vi "create_node.vi"(0 "text":string, 5 "metadatas":cluster{"key":string, "value":string}[](array[cluster]), 7 "vector":dbl[](array[numeric]), 11 "error in":errorcluster) -> (4 "data_node out":refnum<class "data_node.lvclass">, 15 "error out":errorcluster)   [LabVIEW 2020, in "data_node.lvclass"]
uses:
  data_node.lvclass
  data_node.lvclass/data_node.ctl
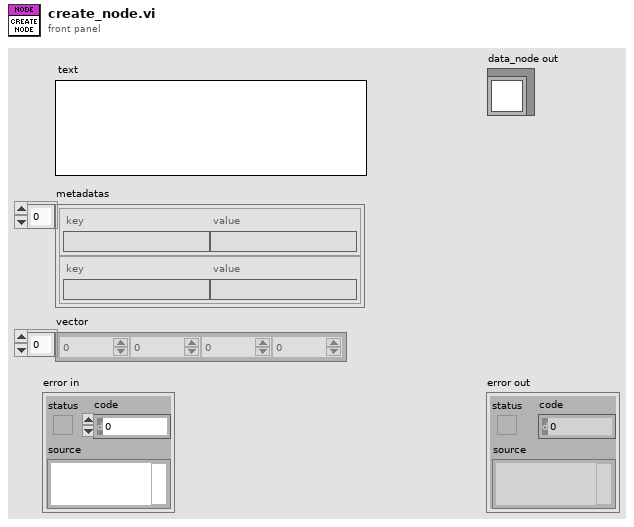
[diagram p1: front panel]
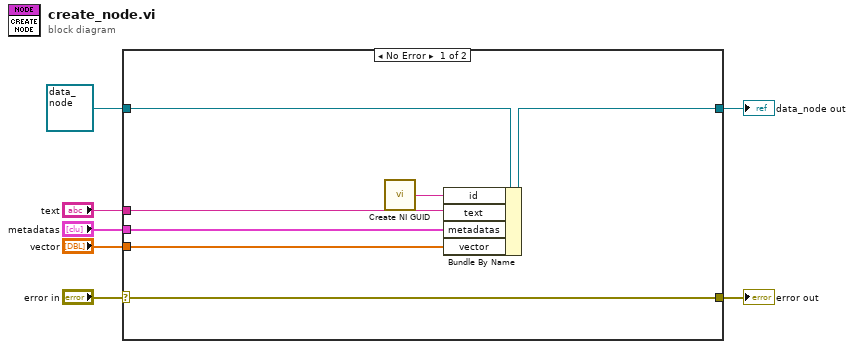
[diagram p0: block diagram]
diagram:
  n1 = case shown="No Error" "error in" {
    selector: "error in" -> [w14 w16]
    tunnel: [w14 w16] -> w6
    tunnel: [w11 w15] -> w4
    tunnel: refnum<class "data_node.lvclass"> refnum ("data_node in") -> [w13 w15]
    tunnel: "text" -> [w10 _]
    tunnel: "metadatas" -> [w9 _]
    tunnel: "vector" -> [w8 _]
    frame No Error {
      n2 = call <vilib>:"Create NI GUID.vi"() -> ("NI GUID"=w12:string)
      n3 = Bundle By Name(cluster=w13, "id"=w12, "text"=w10, "metadatas"=w9, "vector"=w8) -> (w11:refnum<class "data_node.lvclass">)
    }
    frame Error {
    }
  }
  "error out" <- w6
  "data_node out" <- w4
